vi "Configure Measurement.vi"(5 "Display Resolution (6)":dbl=6.0, 6 "Auto Resolution (1: ON)":i32(ring)=1 items=["OFF", "ON", "ONCE"], 7 "Auto Range Value (2.0000000E+2)":dbl=200.0 format="%.7e", 8 "error in (no error)":errorcluster, 9 "Auto Range (1: ON)":i32(ring)=1 items=["OFF", "ON", "ONCE"], 10 "Measurement Function (0: Voltage)":i32(ring) items=["Voltage", "Current", "Resistance", "Charge"], 11 "VISA resource name":refnum<visa-resource-name>) -> (0 "error out":errorcluster, 3 "VISA resource name out":refnum<visa-resource-name>)   [LabVIEW 2020, in "Keithley 6517.lvlib"]
doc: "Configures the range and resolution settings for the measurement functions (Voltage, Current, Resistance and Charge).\n\nNote:\n(1)The specified measurement should be enabled from <b>Configure Measurement Function.vi</b>.\n(2) <B>Display Resolution</B> and <B>Auto Resolution</B> settings are NOT available for <B>model 6514</B>."
uses:
  <instrlib>/Keithley 6517/Keithley 6517.lvlib
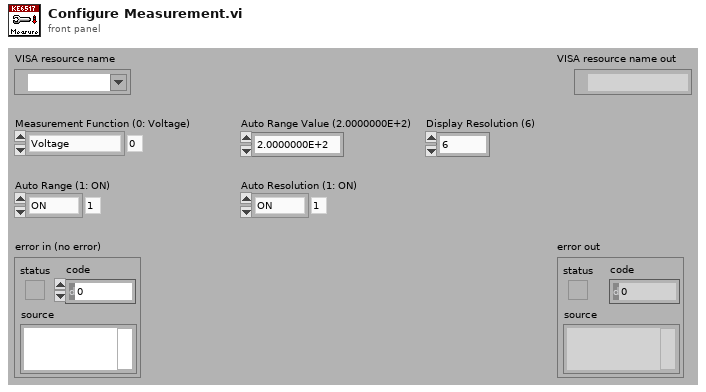
[diagram p1: front panel]
types:
  T1 = typedef "Keithley 6517.lvlib/Extended User Data.ctl" = cluster{"Instrument Model":i32}
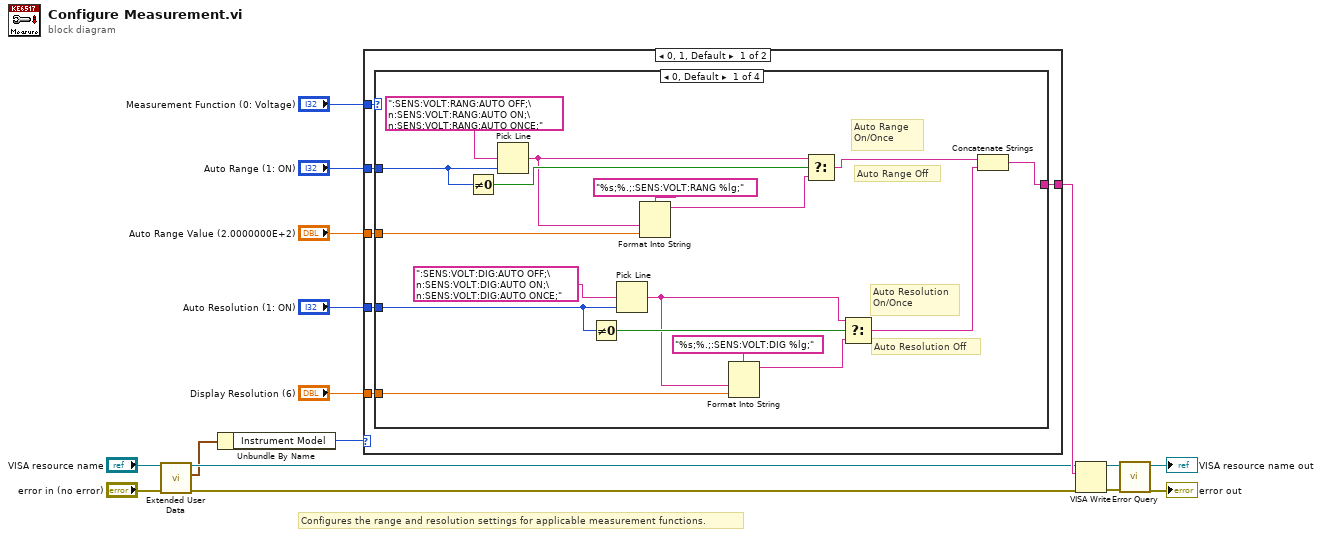
[diagram p0: block diagram]
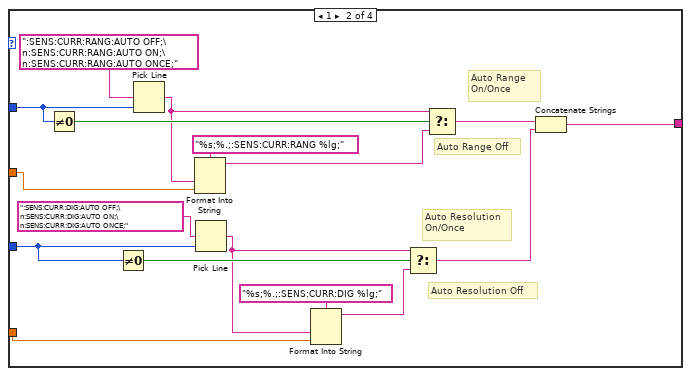
[diagram p2: hidden frame]
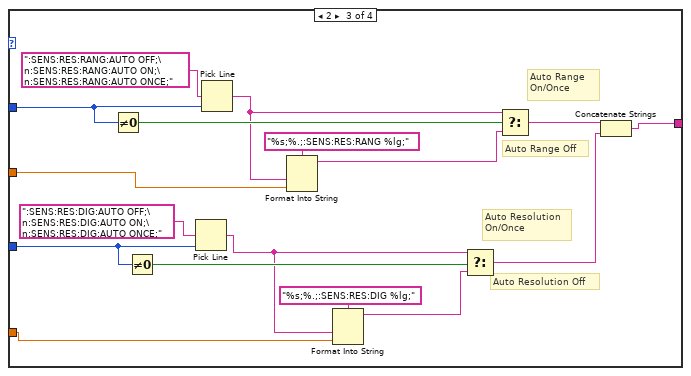
[diagram p3: hidden frame]
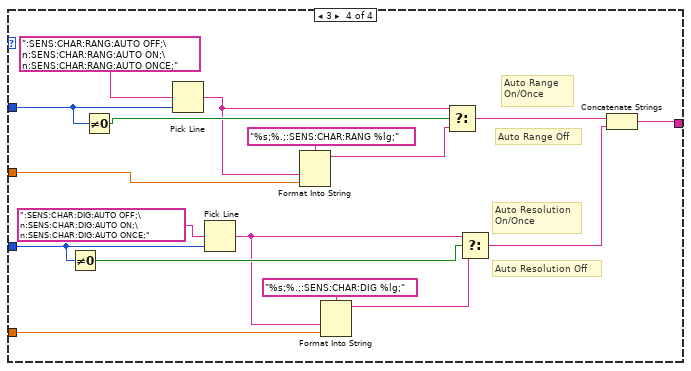
[diagram p4: hidden frame]
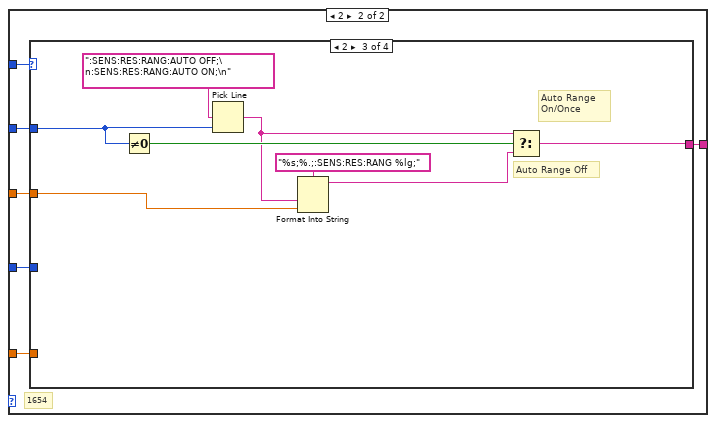
[diagram p5: hidden frame]
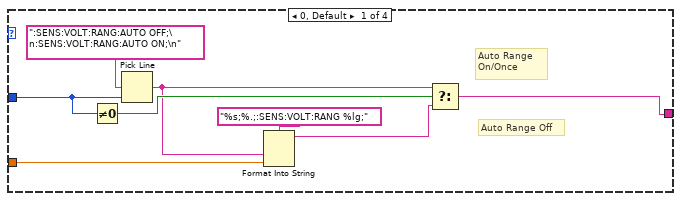
[diagram p6: hidden frame]
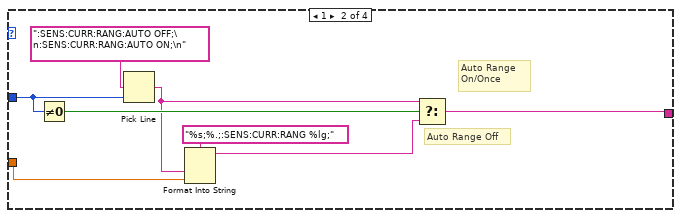
[diagram p7: hidden frame]
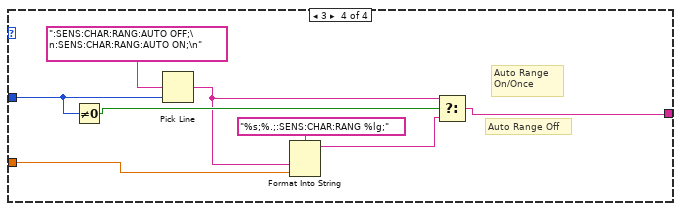
[diagram p8: hidden frame]
diagram:
  # "Configures the range and resolution settings for applicable measurement functions."
  n1 = call <instrlib>:"Extended User Data.vi"("error in (no error)"="error in (no error)", "VISA resource name"="VISA resource name") -> ("error out"=w4:errorcluster, "User Data Out"=w2:T1, "VISA resource name out"=w3:refnum<visa-resource-name>)  [unwired: 7 in]
  n2 = Unbundle By Name(w2) -> ("Instrument Model"=w1:i32)
  n3 = case shown="0, 1, Default" w1 {
    tunnel: "Measurement Function (0: Voltage)" -> [w22 w96]
    tunnel: "Auto Range (1: ON)" -> [w21 w95]
    tunnel: "Auto Range Value (2.0000000E+2)" -> [w20 w94]
    tunnel: "Auto Resolution (1: ON)" -> [w19 w93]
    tunnel: "Display Resolution (6)" -> [w18 w92]
    tunnel: [w17 w91] -> w7
    frame 0, 1, Default {
      n4 = case shown="0, Default" w22 {
        tunnel: w21 -> [w33 w55 w69 w82]
        tunnel: w20 -> [w31 w48 w62 w80]
        tunnel: w19 -> [w28 w54 w66 w77]
        tunnel: w18 -> [w25 w42 w59 w86]
        tunnel: [w34 w44 w63 w83] -> w17
        frame 0, Default {
          # "Auto Resolution Off"
          # "Auto Range Off"
          # "Auto Resolution\nOn/Once"
          # "Auto Range \nOn/Once"
          n5 = Not Equal To 0?(x=w33) -> (x != 0?=w32:bool)
          n6 = Pick Line(multi-line string=":SENS:VOLT:RANG:AUTO OFF;\n:SENS:VOLT:RANG:AUTO ON;\n:SENS:VOLT:RANG:AUTO ONCE;", line index=w33) -> (output string=w30:string)  [unwired: 1 in]
          n7 = Not Equal To 0?(x=w28) -> (x != 0?=w26:bool)
          n8 = Pick Line(multi-line string=":SENS:VOLT:DIG:AUTO OFF;\n:SENS:VOLT:DIG:AUTO ON;\n:SENS:VOLT:DIG:AUTO ONCE;", line index=w28) -> (output string=w24:string)  [unwired: 1 in]
          n9 = Format Into String(format string="%s;%.;:SENS:VOLT:RANG %lg;", w30, w31) -> (resulting string=w29:string)  [unwired: 2 in, 1 out]
          n10 = Format Into String(format string="%s;%.;:SENS:VOLT:DIG %lg;", w24, w25) -> (resulting string=w23:string)  [unwired: 2 in, 1 out]
          n11 = Select(t=w30, s=w32, f=w29) -> (s? t:f=w35:string)
          n12 = Select(t=w24, s=w26, f=w23) -> (s? t:f=w27:string)
          n13 = Concatenate Strings(w35, w27) -> (w34:string)
        }
        frame 1 {
          # "Auto Resolution Off"
          # "Auto Resolution\nOn/Once"
          # "Auto Range Off"
          # "Auto Range \nOn/Once"
          n14 = Not Equal To 0?(x=w55) -> (x != 0?=w53:bool)
          n15 = Not Equal To 0?(x=w54) -> (x != 0?=w50:bool)
          n16 = Pick Line(multi-line string=":SENS:CURR:RANG:AUTO OFF;\n:SENS:CURR:RANG:AUTO ON;\n:SENS:CURR:RANG:AUTO ONCE;", line index=w55) -> (output string=w47:string)  [unwired: 1 in]
          n17 = Format Into String(format string="%s;%.;:SENS:CURR:RANG %lg;", w47, w48) -> (resulting string=w43:string)  [unwired: 2 in, 1 out]
          n18 = Pick Line(multi-line string=":SENS:CURR:DIG:AUTO OFF;\n:SENS:CURR:DIG:AUTO ON;\n:SENS:CURR:DIG:AUTO ONCE;", line index=w54) -> (output string=w41:string)  [unwired: 1 in]
          n19 = Format Into String(format string="%s;%.;:SENS:CURR:DIG %lg;", w41, w42) -> (resulting string=w40:string)  [unwired: 2 in, 1 out]
          n20 = Select(t=w41, s=w50, f=w40) -> (s? t:f=w45:string)
          n21 = Select(t=w47, s=w53, f=w43) -> (s? t:f=w52:string)
          n22 = Concatenate Strings(w52, w45) -> (w44:string)
        }
        frame 2 {
          # "Auto Resolution Off"
          # "Auto Resolution\nOn/Once"
          # "Auto Range Off"
          # "Auto Range \nOn/Once"
          n23 = Not Equal To 0?(x=w69) -> (x != 0?=w68:bool)
          n24 = Not Equal To 0?(x=w66) -> (x != 0?=w65:bool)
          n25 = Pick Line(multi-line string=":SENS:RES:DIG:AUTO OFF;\n:SENS:RES:DIG:AUTO ON;\n:SENS:RES:DIG:AUTO ONCE;", line index=w66) -> (output string=w58:string)  [unwired: 1 in]
          n26 = Pick Line(multi-line string=":SENS:RES:RANG:AUTO OFF;\n:SENS:RES:RANG:AUTO ON;\n:SENS:RES:RANG:AUTO ONCE;", line index=w69) -> (output string=w61:string)  [unwired: 1 in]
          n27 = Format Into String(format string="%s;%.;:SENS:RES:RANG %lg;", w61, w62) -> (resulting string=w60:string)  [unwired: 2 in, 1 out]
          n28 = Format Into String(format string="%s;%.;:SENS:RES:DIG %lg;", w58, w59) -> (resulting string=w57:string)  [unwired: 2 in, 1 out]
          n29 = Select(t=w58, s=w65, f=w57) -> (s? t:f=w64:string)
          n30 = Select(t=w61, s=w68, f=w60) -> (s? t:f=w67:string)
          n31 = Concatenate Strings(w67, w64) -> (w63:string)
        }
        frame 3 {
          # "Auto Resolution Off"
          # "Auto Resolution\nOn/Once"
          # "Auto Range Off"
          # "Auto Range \nOn/Once"
          n32 = Not Equal To 0?(x=w77) -> (x != 0?=w76:bool)
          n33 = Not Equal To 0?(x=w82) -> (x != 0?=w81:bool)
          n34 = Pick Line(multi-line string=":SENS:CHAR:RANG:AUTO OFF;\n:SENS:CHAR:RANG:AUTO ON;\n:SENS:CHAR:RANG:AUTO ONCE;", line index=w82) -> (output string=w79:string)  [unwired: 1 in]
          n35 = Pick Line(multi-line string=":SENS:CHAR:DIG:AUTO OFF;\n:SENS:CHAR:DIG:AUTO ON;\n:SENS:CHAR:DIG:AUTO ONCE;", line index=w77) -> (output string=w75:string)  [unwired: 1 in]
          n36 = Format Into String(format string="%s;%.;:SENS:CHAR:RANG %lg;", w79, w80) -> (resulting string=w78:string)  [unwired: 2 in, 1 out]
          n37 = Format Into String(format string="%s;%.;:SENS:CHAR:DIG %lg;", w75, w86) -> (resulting string=w74:string)  [unwired: 2 in, 1 out]
          n38 = Select(t=w79, s=w81, f=w78) -> (s? t:f=w85:string)
          n39 = Select(t=w75, s=w76, f=w74) -> (s? t:f=w84:string)
          n40 = Concatenate Strings(w85, w84) -> (w83:string)
        }
      }
    }
    frame 2 {
      # "1654"
      n41 = case shown="2" w96 {
        tunnel: w95 -> [w102 w111 w118 w126]
        tunnel: w94 -> [w100 w108 w116 w124]
        tunnel: w93 -> [_ _ _ _]
        tunnel: w92 -> [_ _ _ _]
        tunnel: [w97 w105 w113 w121] -> w91
        frame 0, Default {
          # "Auto Range Off"
          # "Auto Range \nOn/Once"
          n42 = Not Equal To 0?(x=w102) -> (x != 0?=w101:bool)
          n43 = Pick Line(multi-line string=":SENS:VOLT:RANG:AUTO OFF;\n:SENS:VOLT:RANG:AUTO ON;\n", line index=w102) -> (output string=w99:string)  [unwired: 1 in]
          n44 = Format Into String(format string="%s;%.;:SENS:VOLT:RANG %lg;", w99, w100) -> (resulting string=w98:string)  [unwired: 2 in, 1 out]
          n45 = Select(t=w99, s=w101, f=w98) -> (s? t:f=w97:string)
        }
        frame 1 {
          # "Auto Range Off"
          # "Auto Range \nOn/Once"
          n46 = Not Equal To 0?(x=w111) -> (x != 0?=w110:bool)
          n47 = Pick Line(multi-line string=":SENS:CURR:RANG:AUTO OFF;\n:SENS:CURR:RANG:AUTO ON;\n", line index=w111) -> (output string=w107:string)  [unwired: 1 in]
          n48 = Format Into String(format string="%s;%.;:SENS:CURR:RANG %lg;", w107, w108) -> (resulting string=w106:string)  [unwired: 2 in, 1 out]
          n49 = Select(t=w107, s=w110, f=w106) -> (s? t:f=w105:string)
        }
        frame 2 {
          # "Auto Range Off"
          # "Auto Range \nOn/Once"
          n50 = Not Equal To 0?(x=w118) -> (x != 0?=w117:bool)
          n51 = Pick Line(multi-line string=":SENS:RES:RANG:AUTO OFF;\n:SENS:RES:RANG:AUTO ON;\n", line index=w118) -> (output string=w115:string)  [unwired: 1 in]
          n52 = Format Into String(format string="%s;%.;:SENS:RES:RANG %lg;", w115, w116) -> (resulting string=w114:string)  [unwired: 2 in, 1 out]
          n53 = Select(t=w115, s=w117, f=w114) -> (s? t:f=w113:string)
        }
        frame 3 {
          # "Auto Range Off"
          # "Auto Range \nOn/Once"
          n54 = Not Equal To 0?(x=w126) -> (x != 0?=w125:bool)
          n55 = Pick Line(multi-line string=":SENS:CHAR:RANG:AUTO OFF;\n:SENS:CHAR:RANG:AUTO ON;\n", line index=w126) -> (output string=w123:string)  [unwired: 1 in]
          n56 = Format Into String(format string="%s;%.;:SENS:CHAR:RANG %lg;", w123, w124) -> (resulting string=w122:string)  [unwired: 2 in, 1 out]
          n57 = Select(t=w123, s=w125, f=w122) -> (s? t:f=w121:string)
        }
      }
    }
  }
  n58 = VISA Write(VISA resource name=w3, write buffer=w7, error in (no error)=w4) -> (VISA resource name out=w16:refnum<visa-resource-name>, error out=w15:errorcluster)  [unwired: 1 out]
  n59 = call <instrlib>:"Error Query.vi"("error in (no error)"=w15, "VISA resource name"=w16) -> ("error out"=→"error out":errorcluster, "VISA resource name out"=→"VISA resource name out":refnum<visa-resource-name>)  [unwired: 6 in, 2 out]
